vi "Read Number from String Array.vi"(2 "error in (no error)":errorcluster, 3 "Variables":string[](array[string]), 4 "Name":string) -> (0 "error out":errorcluster, 1 "number":dbl)   [LabVIEW 2014]
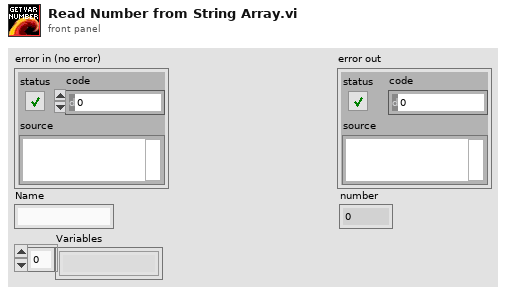
[diagram p1: front panel]
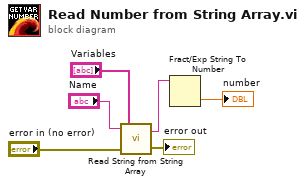
[diagram p0: block diagram]
diagram:
  n1 = call "Read String from String Array.vi"("error in (no error)"="error in (no error)", "Variables"="Variables", "Name"="Name") -> ("error out"=→"error out":errorcluster, "Variable"=w3:string)
  n2 = Fract/Exp String To Number(string=w3) -> (number=→"number":dbl)  [unwired: 3 in, 1 out]
